vi "[FGV] State Calling Info.vi"(0 "Queue Info Set":T1, 1 "error in (no error)":errorcluster, 6 "Action":T3(ring), 8 "Size":i32=128) -> (12 "Queue Info.Get.Current State":T1, 14 "Queue Info.Get.Prev Record":T2(array[cluster]), 15 "error out":errorcluster)   [LabVIEW 2019, in "Template.lvlib"]
uses:
  Template.lvlib
panel:
  out "Queue Info.Ref.Get Current State":T1
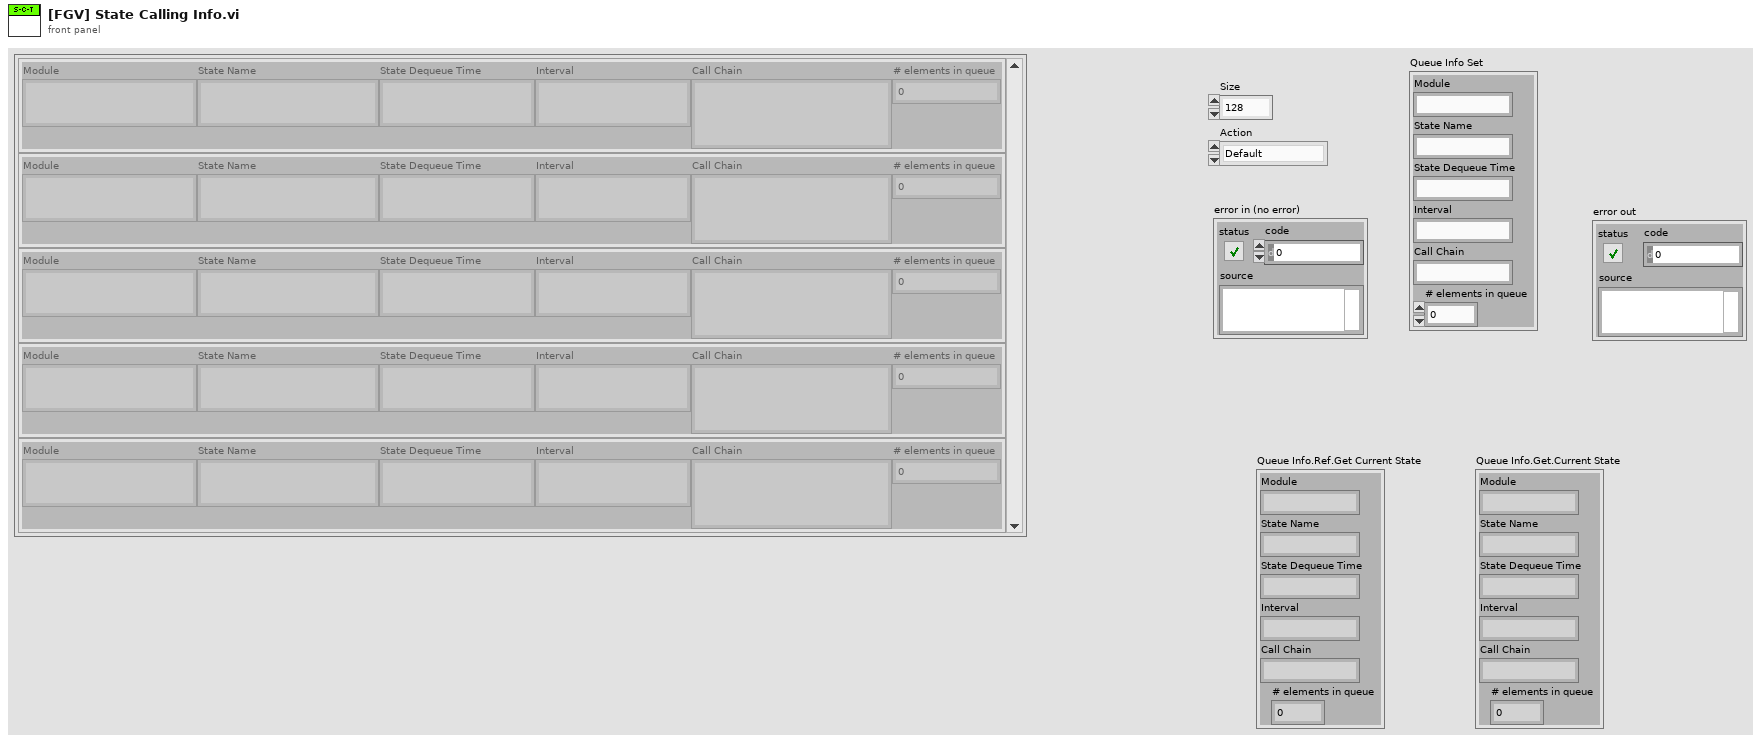
[diagram p1: front panel]
types:
  T1 = cluster{"Module":string, "State Name":string, "State Dequeue Time":string, "Interval":string, "Call Chain":string, "# elements in queue":i32}
  T2 = cluster{"Module":string, "State Name":string, "State Dequeue Time":string, "Interval":string, "Call Chain":string, "# elements in queue":i32}[]
  T3 = enum16{"Default", "Show FP", "Hide FP", "New Data", "Get Data"}
  T4 = enum32{"Invalid", "Standard", "Closed", "Hidden", "Minimized", "Maximized"}
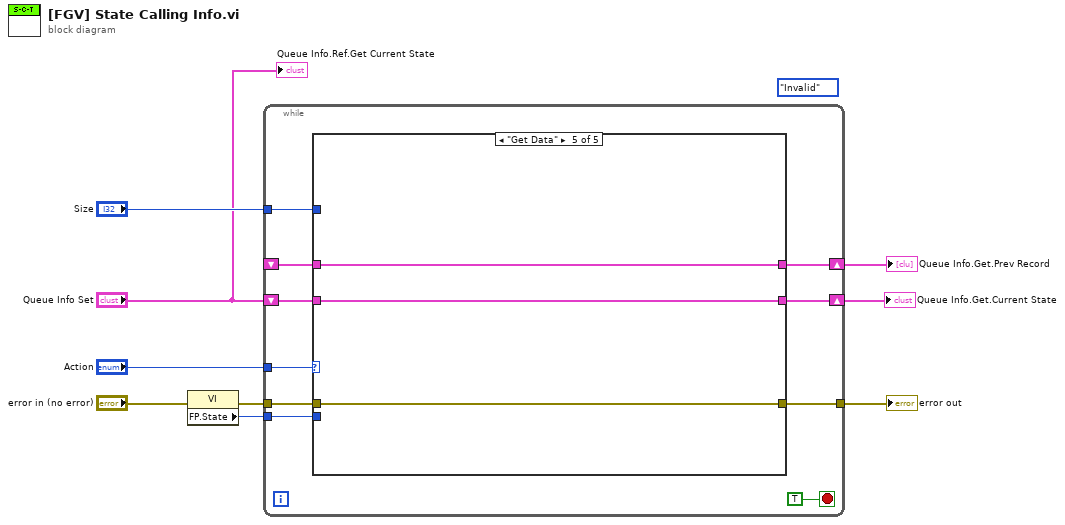
[diagram p0: block diagram]
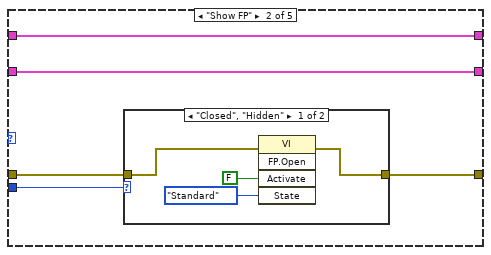
[diagram p3: hidden frame]
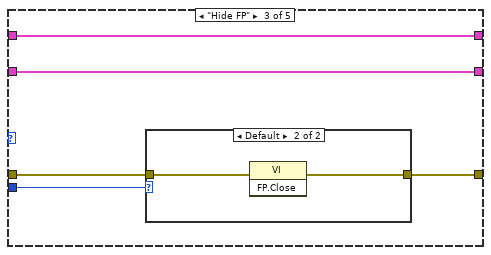
[diagram p5: hidden frame]
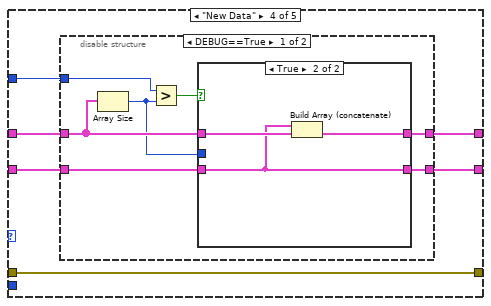
[diagram p7: hidden frame]
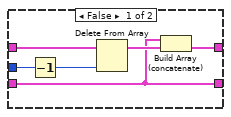
[diagram p8: hidden frame]
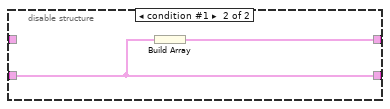
[diagram p9: hidden frame]
diagram:
  (unwired) T4."Invalid" ("Front Panel Window:State")
  n1 = property class="VI"(error in="error in (no error)") -> (error out=w6:errorcluster, "FP.State"=w5:T4)  [unwired: 1 in, 1 out]
  n2 = while {
    tunnel: "Action" -> [w18]
    tunnel: w6 -> [w17]
    tunnel: [w16] -> w8
    shift-right: [w15] -> w4
    shift-left: _ -> [w14]
    tunnel: w5 -> [w12]
    tunnel: "Size" -> [w11]
    shift-right: [w10] -> w1
    shift-left: "Queue Info Set" -> [w13]
    stop <- TRUE stop-if-true
    n3 = case shown="\"Get Data\"" w18 {
      tunnel: w17 -> [w22 w27 w37 w46 w67]
      tunnel: [w22 w26 w36 w46 w67] -> w16
      tunnel: [w21 w25 w35 w44 w66] -> w15
      tunnel: w14 -> [w21 w25 w35 w42 w66]
      tunnel: w13 -> [w20 w23 w33 w43 w65]
      tunnel: w12 -> [_ w24 w34 _ _]
      tunnel: w11 -> [_ _ _ w45 _]
      tunnel: [w20 w23 w33 w41 w65] -> w10
      frame "Default" {
      }
      frame "Show FP" {
        n4 = case shown="\"Closed\", \"Hidden\"" w24 {
          tunnel: w27 -> [w29 w32]
          tunnel: [w28 w32] -> w26
          frame "Closed", "Hidden" {
            n5 = invoke class="VI" method="FP.Open"(error in=w29, "Activate"=FALSE ("Activate?"), "State"=T4."Standard") -> (error out=w28:errorcluster)  [unwired: 2 in, 4 out]
          }
          frame Default {
          }
        }
      }
      frame "Hide FP" {
        n6 = case shown="Default" w34 {
          tunnel: w37 -> [w38 w40]
          tunnel: [w38 w39] -> w36
          frame "Invalid", "Closed" {
          }
          frame Default {
            n7 = invoke class="VI" method="FP.Close"(error in=w40) -> (error out=w39:errorcluster)  [unwired: 2 in, 2 out]
          }
        }
      }
      frame "New Data" {
        n8 = disable-structure shown="DEBUG==True" {
          disable-tunnel: w45 -> [w52 _]
          disable-tunnel: [w51 w64] -> w44
          disable-tunnel: w43 -> [w50 w63]
          disable-tunnel: w42 -> [w49 _]
          disable-tunnel: [w47 w63] -> w41
          frame condition #0 (active) {
            n9 = Array Size(array=w49) -> (size(s)=w48:i32)
            n10 = Greater?(x=w52, y=w48) -> (0:w53:bool)
            n11 = case shown="True" w53 {
              tunnel: [w57 w61] -> w51
              tunnel: w50 -> [w54 w60]
              tunnel: w49 -> [w59 w62]
              tunnel: w48 -> [w56 _]
              tunnel: [w54 w60] -> w47
              frame False {
                n12 = Decrement(x=w56) -> (x-1=w55:i32)
                n13 = Delete From Array(array=w59, index=w55) -> (array with subset deleted=w58:T2)  [unwired: 1 in, 1 out]
                n14 = Build Array (concatenate)(w54, w58) -> (w57:T2)
              }
              frame True {
                n15 = Build Array (concatenate)(w60, w62) -> (w61:T2)
              }
            }
          }
          frame condition #1 {
            n16 = Build Array(w63) -> (w64:T2)
          }
        }
      }
      frame "Get Data" {
      }
    }
  }
  "error out" <- w8
  "Queue Info.Get.Prev Record" <- w4
  "Queue Info.Get.Current State" <- w1
  "Queue Info.Ref.Get Current State" <- "Queue Info Set"
